vi "ProcessBScan.vi"(0 "data":dbl[][](array[numeric]), 1 "Image Avg 2D":dbl, 2 "Doppler 2D":bool, 5 "zero array":dbl[][](array[numeric]), 7 "lambdaCalArray":dbl[](array[numeric]), 9 "FFTW3 Arrays":T1={"data_points"=0, "camera_pixel"=2048, "zero array"=[], "complex zero array"=[]}, 12 "Power 2D":dbl, 13 "Period":dbl) -> (4 "Image":dbl[][](array[numeric]), 6 "buffer out":dbl[][](array[numeric]), 10 "velocity_profile":dbl[][](array[numeric]), 15 "error out":errorcluster)   [LabVIEW 2017]
uses:
  development-testing/SoftwareObjects/ConfigProcessing/ConfigProcessing.lvclass
  classes/HardwareObjects/Spectrometer/Spectrometer.lvclass
panel:
  in  "Processing Settings":refnum<class "ConfigProcessing.lvclass">
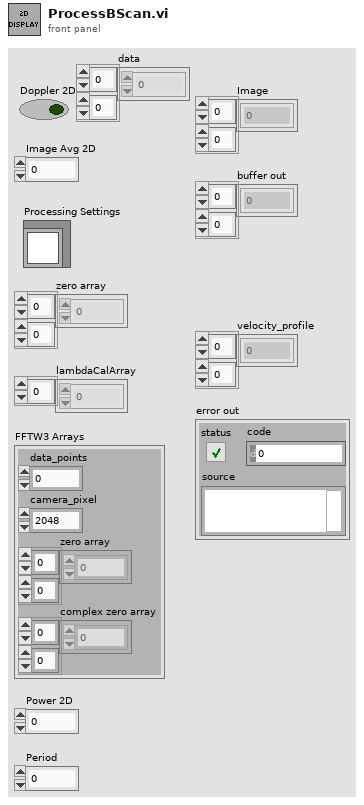
[diagram p1: front panel]
types:
  T1 = cluster{"data_points":i32, "camera_pixel":i32, "zero array":dbl[][], "complex zero array":dbl[][]}
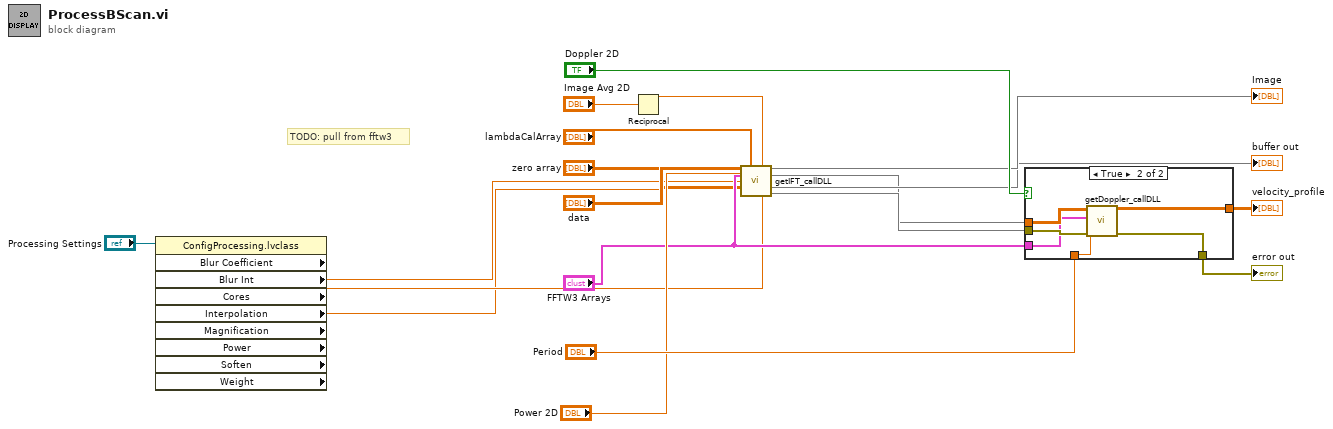
[diagram p0: block diagram]
diagram:
  # "TODO: pull from fftw3"
  n1 = property class="ConfigProcessing.lvclass" props=["Blur Coefficient", "Blur Int", "Cores", "Interpolation", "Magnification", "Power", "Soften", "Weight"](reference="Processing Settings") -> ("Blur Int"=w8:dbl, "Cores"=w6:dbl, "Interpolation"=w5:dbl)  [unwired: 1 in, 7 out]
  n2 = Reciprocal(x="Image Avg 2D") -> (1/x=w14:dbl)
  n3 = call "getIFT_callDLL.vi"(0:"data", 1:"lambdaCalArray", 2:"Power 2D", 3:w14, 5:"FFTW3 Arrays", 7:w8, 9:"zero array", 12:w5, 14:w6) -> (4:→"Image", 6:w1, 10:→"buffer out", 15:w4)  [unwired: 3 in]
  n4 = case shown="True" "Doppler 2D" {
    tunnel: "FFTW3 Arrays" -> [_ w23]
    tunnel: w4 -> [w21 w27]
    tunnel: [w21 w26] -> w15
    tunnel: w1 -> [w20 w25]
    tunnel: "Period" -> [_ w24]
    tunnel: [w20 w22] -> w17
    frame False {
    }
    frame True {
      n5 = call "getDoppler_callDLL.vi"("Error in"=w27, "Spectrometer.lvclass"=w24, "Processing Settings"=w23, "Data_complex"=w25) -> ("error out"=w26:errorcluster, "velocity_profile"=w22:dbl[][])  [unwired: 6 in]
    }
  }
  "velocity_profile" <- w17
  "error out" <- w15
